vi "temp comprasion.vi"(9 "Upper Limit":dbl[](array[numeric]), 10 "Array":dbl[](array[numeric]), 11 "Ambient temp":dbl) -> (1 "output array":bool[](array[boolean]), 2 "pass or fail":T1(array[cluster]), 3 "temp array":dbl[](array[numeric]))   [LabVIEW 2021]
uses:
  controls/comparison selection.ctl
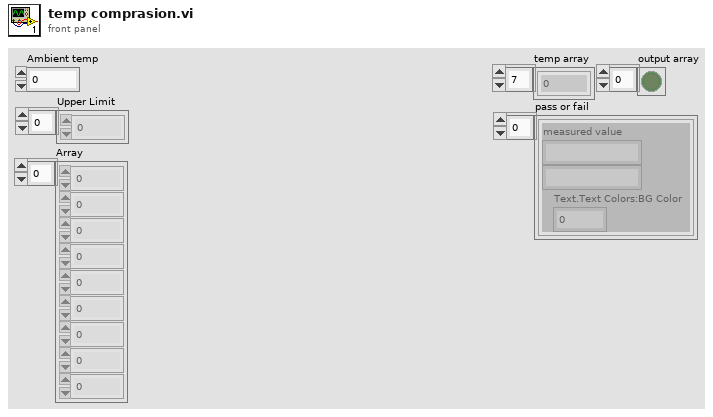
[diagram p1: front panel]
types:
  T1 = cluster{"measured value":string, string, "Text.Text Colors:BG Color":u32}[]
  T2 = typedef "comparison selection.ctl" = enum16{"None", "in-range?", "less than?", "greater than?", "equal to?", "not equal to?", "less or equal to?", "greater or equal to?"}
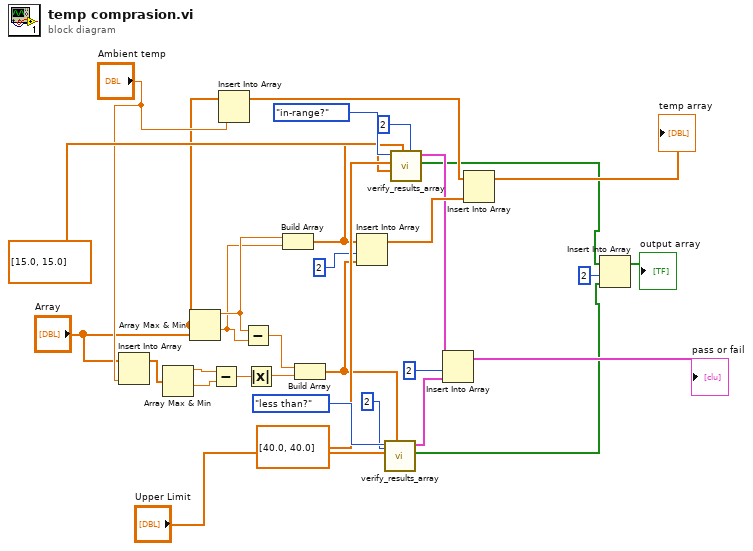
[diagram p0: block diagram]
diagram:
  n1 = Insert Into Array(array="Array", new element="Ambient temp") -> (w3:dbl[])  [unwired: 1 in]
  n2 = Array Max & Min(array=w3) -> (max value=w5:dbl, min value=w6:dbl)  [unwired: 2 out]
  n3 = Array Max & Min(array="Array") -> (max value=w25:dbl, min value=w24:dbl)  [unwired: 2 out]
  n4 = Subtract(x=w5, y=w6) -> (x-y=w31:dbl)
  n5 = Insert Into Array(array="Array", new element="Ambient temp") -> (w28:dbl[])  [unwired: 1 in]
  n6 = Subtract(x=w25, y=w24) -> (x-y=w30:dbl)
  n7 = Absolute Value(x=w31) -> (abs(x)=w7:dbl)
  n8 = Build Array(w25, w24) -> (w19:dbl[])
  n9 = Build Array(w30, w7) -> (w15:dbl[])
  n10 = Insert Into Array(array=w19, index=2, new element=w15) -> (w21:dbl[])
  n11 = call "verify_results_array.vi"("precision (6)"=i16 2, "Mesured values"=w15, "Upper Limit"="Upper Limit", "comparison"=comparison_selection."less than?") -> ("Pass or fail array"=w10:bool[], "Array"=w17:T1)  [unwired: 5 in, 1 out]
  n12 = call "verify_results_array.vi"("precision (6)"=i16 2, "Mesured values"=w19, "Lower Limit"=dbl[] [15.0, 15.0], "Upper Limit"=dbl[] [40.0, 40.0], "comparison"=comparison_selection."in-range?") -> ("Pass or fail array"=w11:bool[], "Array"=w18:T1)  [unwired: 4 in, 1 out]
  n13 = Insert Into Array(array=w18, index=2, new element=w17) -> (→"pass or fail":T1)
  n14 = Insert Into Array(array=w28, new element=w21) -> (→"temp array":dbl[])  [unwired: 1 in]
  n15 = Insert Into Array(array=w11, index=2, new element=w10) -> (→"output array":bool[])
